vi "mules_number2zeroedstr.vi"(1 "minNumberDigits":i32=2, 2 "number":i32) -> (0 "string":string)   [LabVIEW 2013]
doc: "cambia le agrega un cero a la izquerda a los numero menores a 10"
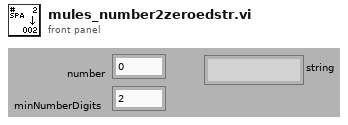
[diagram p1: front panel]
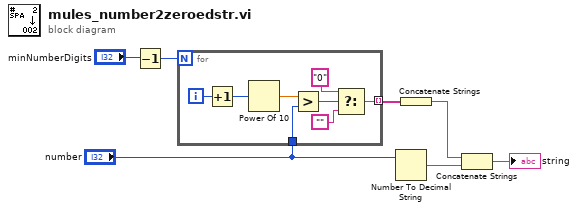
[diagram p0: block diagram]
diagram:
  n1 = Decrement(x="minNumberDigits") -> (x-1=w1:i32)
  n2 = for {
    N: w1 -> [_]
    tunnel: [w12] -> w5 mode=indexing
    tunnel: "number" -> [w11]
    i -> [w9]
    n3 = Increment(x=w9) -> (x+1=w8:i32)
    n4 = Power Of 10(x=w8) -> (10^x=w10:dbl)
    n5 = Greater?(x=w10, y=w11) -> (0:w14:bool)
    n6 = Select(t="0", s=w14, f="") -> (s? t:f=w12:string)
  }
  n7 = Number To Decimal String(number="number") -> (decimal integer string=w7:string)  [unwired: 1 out]
  n8 = Concatenate Strings(w5) -> (w3:string)
  n9 = Concatenate Strings(w3, w7) -> (→"string":string)
